vi "Make Defect Pair (old).vi"() -> ()   [LabVIEW 2010]
uses:
  <vilib>/Analysis/NI_AALPro.lvlib
  <vilib>/Analysis/_algsub.llb/Real Vector Norm.vi
panel:
  out "Atoms to Add":cluster{"Species":string, "Position":dbl[]}[](array[cluster])
  out "Atoms to remove":T1(array[cluster])
  out "Defected Structure":T2={"Structure Name"="Gamma8_64atom", "Lattice vector a"=[13.21796569573, 0.0, 0.0], "Lattice vector b"=[0.0, 13.21796569573, 0.0], "Lattice vector c"=[0.0, 0.0, 13.21796569573], "Atoms Array"=[{"Atom Name"="Cd", "Positions (Direct)"=[[0.0, 0.0, 0.0], [0.0, 0.0, 0.5], [0.0, 0.5, 0.0], [0.0, 0.5, 0.5], [0.5, 0.0, 0.0], [0.5, 0.0, 0.5], [0.5, 0.5, 0.0], [0.5, 0.5, 0.5], [0.0, 0.25, 0.25], [0.0, 0.25, 0.75], [0.0, 0.75, 0.25], [0.0, 0.75, 0.75], [0.5, 0.25, 0.25], [0.5, 0.25, 0.75], [0.5, 0.75, 0.25], [0.5, 0.75, 0.75], [0.25, 0.0, 0.25], [0.25, 0.0, 0.75], [0.25, 0.5, 0.25], [0.25, 0.5, 0.75], [0.75, 0.0, 0.25], [0.75, 0.0, 0.75], [0.75, 0.5, 0.25], [0.75, 0.5, 0.75], [0.25, 0.25, 0.0], [0.25, 0.25, 0.5], [0.25, 0.75, 0.0], [0.25, 0.75, 0.5], [0.75, 0.25, 0.0], [0.75, 0.25, 0.5], [0.75, 0.75, 0.0], [0.75, 0.75, 0.5]], "Positions (Cartesian)"=[[0.0, 0.0, 0.0], [0.0, 0.0, 6.608982847865], [0.0, 6.608982847865, 0.0], [0.0, 6.608982847865, 6.608982847865], [6.608982847865, 0.0, 0.0], [6.608982847865, 0.0, 6.608982847865], [6.608982847865, 6.608982847865, 0.0], [6.608982847865, 6.608982847865, 6.608982847865], [0.0, 3.3044914239325, 3.3044914239325], [0.0, 3.3044914239325, 9.913474271797499], [0.0, 9.913474271797499, 3.3044914239325], [0.0, 9.913474271797499, 9.913474271797499], [6.608982847865, 3.3044914239325, 3.3044914239325], [6.608982847865, 3.3044914239325, 9.913474271797499], [6.608982847865, 9.913474271797499, 3.3044914239325], [6.608982847865, 9.913474271797499, 9.913474271797499], [3.3044914239325, 0.0, 3.3044914239325], [3.3044914239325, 0.0, 9.913474271797499], [3.3044914239325, 6.608982847865, 3.3044914239325], [3.3044914239325, 6.608982847865, 9.913474271797499], [9.913474271797499, 0.0, 3.3044914239325], [9.913474271797499, 0.0, 9.913474271797499], [9.913474271797499, 6.608982847865, 3.3044914239325], [9.913474271797499, 6.608982847865, 9.913474271797499], [3.3044914239325, 3.3044914239325, 0.0], [3.3044914239325, 3.3044914239325, 6.608982847865], [3.3044914239325, 9.913474271797499, 0.0], [3.3044914239325, 9.913474271797499, 6.608982847865], [9.913474271797499, 3.3044914239325, 0.0], [9.913474271797499, 3.3044914239325, 6.608982847865], [9.913474271797499, 9.913474271797499, 0.0], [9.913474271797499, 9.913474271797499, 6.608982847865]]}, {"Atom Name"="Te", "Positions (Direct)"=[[0.125, 0.125, 0.125], [0.125, 0.125, 0.625], [0.125, 0.625, 0.125], [0.125, 0.625, 0.625], [0.625, 0.125, 0.125], [0.625, 0.125, 0.625], [0.625, 0.625, 0.125], [0.625, 0.625, 0.625], [0.375, 0.375, 0.125], [0.375, 0.375, 0.625], [0.375, 0.875, 0.125], [0.375, 0.875, 0.625], [0.875, 0.375, 0.125], [0.875, 0.375, 0.625], [0.875, 0.875, 0.125], [0.875, 0.875, 0.625], [0.375, 0.125, 0.375], [0.375, 0.125, 0.875], [0.375, 0.625, 0.375], [0.375, 0.625, 0.875], [0.875, 0.125, 0.375], [0.875, 0.125, 0.875], [0.875, 0.625, 0.375], [0.875, 0.625, 0.875], [0.125, 0.375, 0.375], [0.125, 0.375, 0.875], [0.125, 0.875, 0.375], [0.125, 0.875, 0.875], [0.625, 0.375, 0.375], [0.625, 0.375, 0.875], [0.625, 0.875, 0.375], [0.625, 0.875, 0.875]], "Positions (Cartesian)"=[[1.65224571196625, 1.65224571196625, 1.65224571196625], [1.65224571196625, 1.65224571196625, 8.261228559831249], [1.65224571196625, 8.261228559831249, 1.65224571196625], [1.65224571196625, 8.261228559831249, 8.261228559831249], [8.261228559831249, 1.65224571196625, 1.65224571196625], [8.261228559831249, 1.65224571196625, 8.261228559831249], [8.261228559831249, 8.261228559831249, 1.65224571196625], [8.261228559831249, 8.261228559831249, 8.261228559831249], [4.9567371358987495, 4.9567371358987495, 1.65224571196625], [4.9567371358987495, 4.9567371358987495, 8.261228559831249], [4.9567371358987495, 11.56571998376375, 1.65224571196625], [4.9567371358987495, 11.56571998376375, 8.261228559831249], [11.56571998376375, 4.9567371358987495, 1.65224571196625], [11.56571998376375, 4.9567371358987495, 8.261228559831249], [11.56571998376375, 11.56571998376375, 1.65224571196625], [11.56571998376375, 11.56571998376375, 8.261228559831249], [4.9567371358987495, 1.65224571196625, 4.9567371358987495], [4.9567371358987495, 1.65224571196625, 11.56571998376375], [4.9567371358987495, 8.261228559831249, 4.9567371358987495], [4.9567371358987495, 8.261228559831249, 11.56571998376375], [11.56571998376375, 1.65224571196625, 4.9567371358987495], [11.56571998376375, 1.65224571196625, 11.56571998376375], [11.56571998376375, 8.261228559831249, 4.9567371358987495], [11.56571998376375, 8.261228559831249, 11.56571998376375], [1.65224571196625, 4.9567371358987495, 4.9567371358987495], [1.65224571196625, 4.9567371358987495, 11.56571998376375], [1.65224571196625, 11.56571998376375, 4.9567371358987495], [1.65224571196625, 11.56571998376375, 11.56571998376375], [8.261228559831249, 4.9567371358987495, 4.9567371358987495], [8.261228559831249, 4.9567371358987495, 11.56571998376375], [8.261228559831249, 11.56571998376375, 4.9567371358987495], [8.261228559831249, 11.56571998376375, 11.56571998376375]]}], "# of atoms"=64}
  out "Defect Options":T3(array[cluster])=[{"Position"=[1.65224571196625, 1.65224571196625, 1.65224571196625], "Distance from 1"=2.8617735197133576, "Index"=0}, {"Position"=[4.9567371358987495, 4.9567371358987495, 1.65224571196625], "Distance from 1"=7.201972088359295, "Index"=8}, {"Position"=[4.9567371358987495, 1.65224571196625, 4.9567371358987495], "Distance from 1"=7.201972088359295, "Index"=16}, {"Position"=[1.65224571196625, 4.9567371358987495, 4.9567371358987495], "Distance from 1"=7.201972088359295, "Index"=24}]
  in  "Defect 2":cluster{"Species":string, "Defect Type":string}={"Species"="Te", "Defect Type"="Vacancy"}
  in  "Defect 1":cluster{"Species":string, "Defect Type":string}={"Species"="Cd", "Defect Type"="Vacancy"}
  in  "Defect 1 Atom Index":i32
  in  "Current Atomic Structure":T2={"Structure Name"="Gamma8_64atom", "Lattice vector a"=[13.21796569573, 0.0, 0.0], "Lattice vector b"=[0.0, 13.21796569573, 0.0], "Lattice vector c"=[0.0, 0.0, 13.21796569573], "Atoms Array"=[{"Atom Name"="Cd", "Positions (Direct)"=[[0.0, 0.0, 0.0], [0.0, 0.0, 0.5], [0.0, 0.5, 0.0], [0.0, 0.5, 0.5], [0.5, 0.0, 0.0], [0.5, 0.0, 0.5], [0.5, 0.5, 0.0], [0.5, 0.5, 0.5], [0.0, 0.25, 0.25], [0.0, 0.25, 0.75], [0.0, 0.75, 0.25], [0.0, 0.75, 0.75], [0.5, 0.25, 0.25], [0.5, 0.25, 0.75], [0.5, 0.75, 0.25], [0.5, 0.75, 0.75], [0.25, 0.0, 0.25], [0.25, 0.0, 0.75], [0.25, 0.5, 0.25], [0.25, 0.5, 0.75], [0.75, 0.0, 0.25], [0.75, 0.0, 0.75], [0.75, 0.5, 0.25], [0.75, 0.5, 0.75], [0.25, 0.25, 0.0], [0.25, 0.25, 0.5], [0.25, 0.75, 0.0], [0.25, 0.75, 0.5], [0.75, 0.25, 0.0], [0.75, 0.25, 0.5], [0.75, 0.75, 0.0], [0.75, 0.75, 0.5]], "Positions (Cartesian)"=[[0.0, 0.0, 0.0], [0.0, 0.0, 6.608982847865], [0.0, 6.608982847865, 0.0], [0.0, 6.608982847865, 6.608982847865], [6.608982847865, 0.0, 0.0], [6.608982847865, 0.0, 6.608982847865], [6.608982847865, 6.608982847865, 0.0], [6.608982847865, 6.608982847865, 6.608982847865], [0.0, 3.3044914239325, 3.3044914239325], [0.0, 3.3044914239325, 9.913474271797499], [0.0, 9.913474271797499, 3.3044914239325], [0.0, 9.913474271797499, 9.913474271797499], [6.608982847865, 3.3044914239325, 3.3044914239325], [6.608982847865, 3.3044914239325, 9.913474271797499], [6.608982847865, 9.913474271797499, 3.3044914239325], [6.608982847865, 9.913474271797499, 9.913474271797499], [3.3044914239325, 0.0, 3.3044914239325], [3.3044914239325, 0.0, 9.913474271797499], [3.3044914239325, 6.608982847865, 3.3044914239325], [3.3044914239325, 6.608982847865, 9.913474271797499], [9.913474271797499, 0.0, 3.3044914239325], [9.913474271797499, 0.0, 9.913474271797499], [9.913474271797499, 6.608982847865, 3.3044914239325], [9.913474271797499, 6.608982847865, 9.913474271797499], [3.3044914239325, 3.3044914239325, 0.0], [3.3044914239325, 3.3044914239325, 6.608982847865], [3.3044914239325, 9.913474271797499, 0.0], [3.3044914239325, 9.913474271797499, 6.608982847865], [9.913474271797499, 3.3044914239325, 0.0], [9.913474271797499, 3.3044914239325, 6.608982847865], [9.913474271797499, 9.913474271797499, 0.0], [9.913474271797499, 9.913474271797499, 6.608982847865]]}, {"Atom Name"="Te", "Positions (Direct)"=[[0.125, 0.125, 0.125], [0.125, 0.125, 0.625], [0.125, 0.625, 0.125], [0.125, 0.625, 0.625], [0.625, 0.125, 0.125], [0.625, 0.125, 0.625], [0.625, 0.625, 0.125], [0.625, 0.625, 0.625], [0.375, 0.375, 0.125], [0.375, 0.375, 0.625], [0.375, 0.875, 0.125], [0.375, 0.875, 0.625], [0.875, 0.375, 0.125], [0.875, 0.375, 0.625], [0.875, 0.875, 0.125], [0.875, 0.875, 0.625], [0.375, 0.125, 0.375], [0.375, 0.125, 0.875], [0.375, 0.625, 0.375], [0.375, 0.625, 0.875], [0.875, 0.125, 0.375], [0.875, 0.125, 0.875], [0.875, 0.625, 0.375], [0.875, 0.625, 0.875], [0.125, 0.375, 0.375], [0.125, 0.375, 0.875], [0.125, 0.875, 0.375], [0.125, 0.875, 0.875], [0.625, 0.375, 0.375], [0.625, 0.375, 0.875], [0.625, 0.875, 0.375], [0.625, 0.875, 0.875]], "Positions (Cartesian)"=[[1.65224571196625, 1.65224571196625, 1.65224571196625], [1.65224571196625, 1.65224571196625, 8.261228559831249], [1.65224571196625, 8.261228559831249, 1.65224571196625], [1.65224571196625, 8.261228559831249, 8.261228559831249], [8.261228559831249, 1.65224571196625, 1.65224571196625], [8.261228559831249, 1.65224571196625, 8.261228559831249], [8.261228559831249, 8.261228559831249, 1.65224571196625], [8.261228559831249, 8.261228559831249, 8.261228559831249], [4.9567371358987495, 4.9567371358987495, 1.65224571196625], [4.9567371358987495, 4.9567371358987495, 8.261228559831249], [4.9567371358987495, 11.56571998376375, 1.65224571196625], [4.9567371358987495, 11.56571998376375, 8.261228559831249], [11.56571998376375, 4.9567371358987495, 1.65224571196625], [11.56571998376375, 4.9567371358987495, 8.261228559831249], [11.56571998376375, 11.56571998376375, 1.65224571196625], [11.56571998376375, 11.56571998376375, 8.261228559831249], [4.9567371358987495, 1.65224571196625, 4.9567371358987495], [4.9567371358987495, 1.65224571196625, 11.56571998376375], [4.9567371358987495, 8.261228559831249, 4.9567371358987495], [4.9567371358987495, 8.261228559831249, 11.56571998376375], [11.56571998376375, 1.65224571196625, 4.9567371358987495], [11.56571998376375, 1.65224571196625, 11.56571998376375], [11.56571998376375, 8.261228559831249, 4.9567371358987495], [11.56571998376375, 8.261228559831249, 11.56571998376375], [1.65224571196625, 4.9567371358987495, 4.9567371358987495], [1.65224571196625, 4.9567371358987495, 11.56571998376375], [1.65224571196625, 11.56571998376375, 4.9567371358987495], [1.65224571196625, 11.56571998376375, 11.56571998376375], [8.261228559831249, 4.9567371358987495, 4.9567371358987495], [8.261228559831249, 4.9567371358987495, 11.56571998376375], [8.261228559831249, 11.56571998376375, 4.9567371358987495], [8.261228559831249, 11.56571998376375, 11.56571998376375]]}], "# of atoms"=64}
  in  "Maximum Distnce":dbl=8.0
  in  "Minimum Distance":dbl
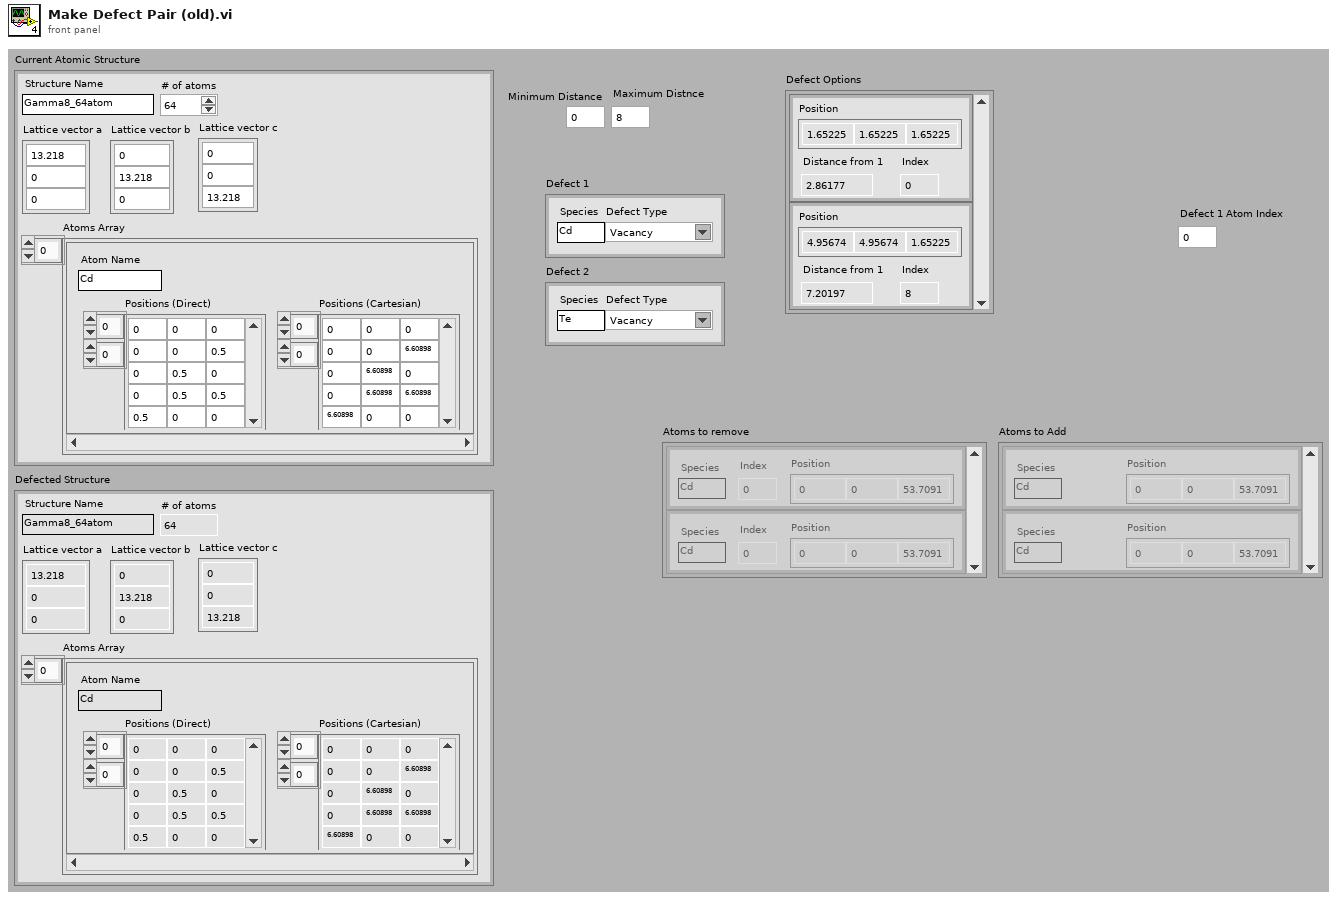
[diagram p1: front panel]
types:
  T1 = cluster{"Species":string, "Index":dbl, "Position":dbl[]}[]
  T2 = cluster{"Structure Name":string, "Lattice vector a":dbl[], "Lattice vector b":dbl[], "Lattice vector c":dbl[], "Atoms Array":cluster{"Atom Name":string, "Positions (Direct)":dbl[][], "Positions (Cartesian)":dbl[][]}[], "# of atoms":i32}
  T3 = cluster{"Position":dbl[], "Distance from 1":dbl, "Index":i32}[]
  T4 = cluster{"Positions (Cartesian)":dbl[], "norm":dbl, i32}[]
  T5 = cluster{"Atom Name":string, "Positions (Direct)":dbl[][], "Positions (Cartesian)":dbl[][]}[]
  T6 = cluster{"Species":string, "Defect 1 Atom Index":i32, "Positions (Cartesian)":dbl[]}
  T7 = cluster{"Atom Name":string, "Defect 1 Atom Index":i32, "Positions (Cartesian)":dbl[]}
  T8 = cluster{"Species":string, "Positions (Cartesian)":dbl[]}
  T9 = cluster{"Positions (Cartesian)":dbl[], "norm":dbl, i32}
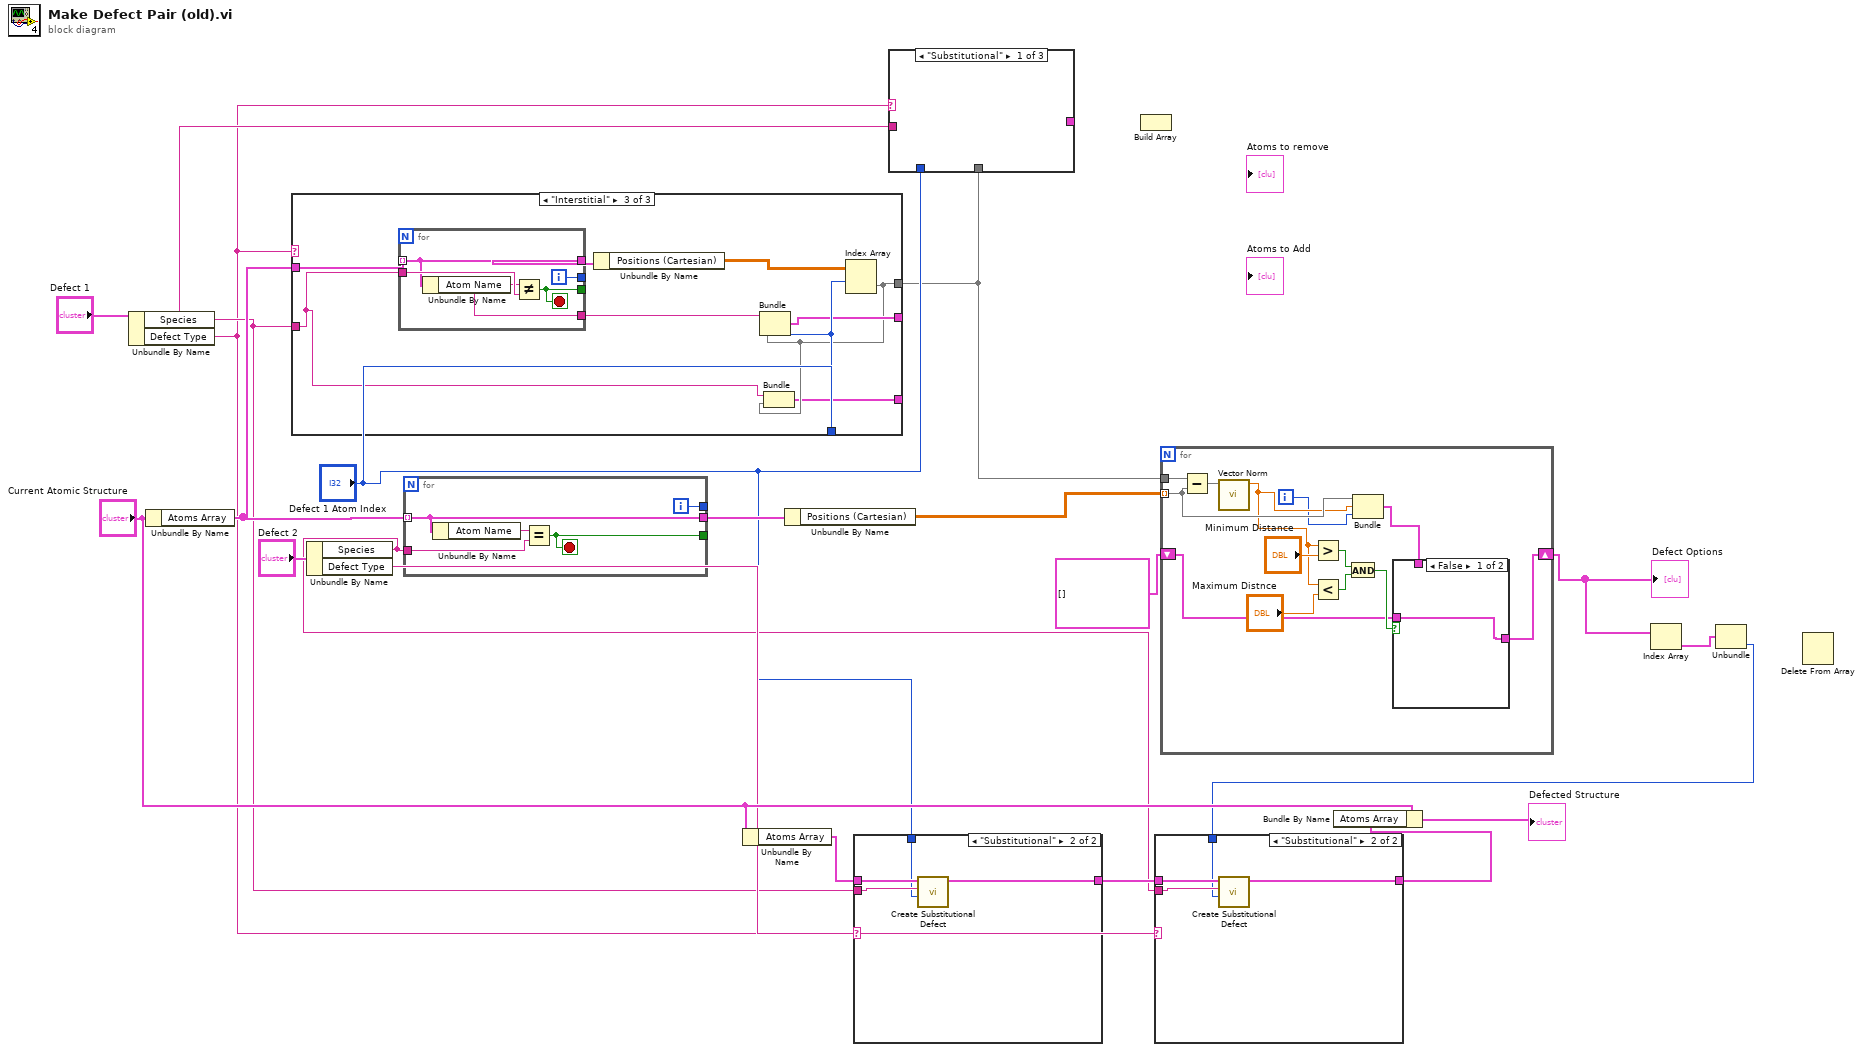
[diagram p0: block diagram]
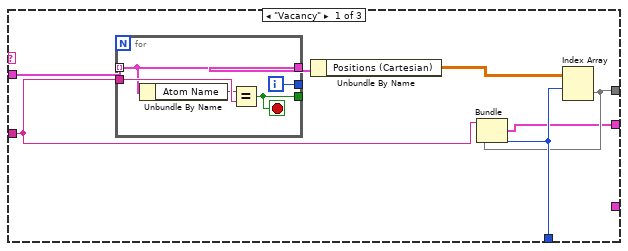
[diagram p2: hidden frame]
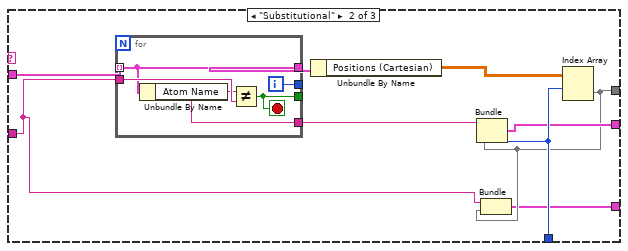
[diagram p3: hidden frame]
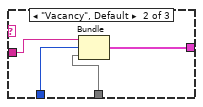
[diagram p4: hidden frame]
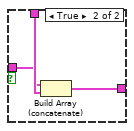
[diagram p8: hidden frame]
diagram:
  n1 = Unbundle By Name("Defect 1") -> ("Species"=w4:string, "Defect Type"=w1:string)
  n2 = Unbundle By Name("Current Atomic Structure") -> ("Atoms Array"=w20:T5)
  n3 = case shown="\"Interstitial\"" w1 {
    tunnel: w20 -> [w27 w41 w55]
    tunnel: w4 -> [w24 w35 w49]
    tunnel: "Defect 1 Atom Index" -> [w23 w38 w52]
    tunnel: [w22 w34 w48] -> w2
    tunnel: [w21 w37 w51] -> _
    tunnel: [_ w33 w47] -> _
    frame "Vacancy" {
      n4 = for {
        tunnel: w27 -> [w28] mode=indexing
        tunnel: w24 -> [w32]
        tunnel: [w30] -> _
        tunnel: [w29] -> _
        tunnel: [w28] -> w26
        i -> [w30]
        stop <- w29 stop-if-true
        n5 = Unbundle By Name(w28) -> ("Atom Name"=w31:string)
        n6 = Equal?(x=w31, y=w32) -> (x = y?=w29:bool)
      }
      n7 = Unbundle By Name(w26) -> ("Positions (Cartesian)"=w25:dbl[][])
      n8 = Index Array(array=w25, index (row)=w23) -> (element=w22:dbl[])  [unwired: 1 in]
      n9 = Bundle("Species"=w24, "Defect 1 Atom Index"=w23, "Positions (Cartesian)"=w22) -> (w21:T6)  [unwired: 1 in]
    }
    frame "Substitutional" {
      n10 = for {
        tunnel: w41 -> [w43] mode=indexing
        tunnel: w35 -> [w46]
        tunnel: [w45] -> _
        tunnel: [w44] -> _
        tunnel: [w43] -> w40
        tunnel: [w42] -> w36
        i -> [w45]
        stop <- w44 stop-if-true
        n11 = Unbundle By Name(w43) -> ("Atom Name"=w42:string)
        n12 = Not Equal?(x=w42, y=w46) -> (x != y?=w44:bool)
      }
      n13 = Unbundle By Name(w40) -> ("Positions (Cartesian)"=w39:dbl[][])
      n14 = Index Array(array=w39, index (row)=w38) -> (element=w34:dbl[])  [unwired: 1 in]
      n15 = Bundle("Atom Name"=w36, "Defect 1 Atom Index"=w38, "Positions (Cartesian)"=w34) -> (w37:T7)  [unwired: 1 in]
      n16 = Bundle("Species"=w35, "Positions (Cartesian)"=w34) -> (w33:T8)  [unwired: 1 in]
    }
    frame "Interstitial" {
      n17 = for {
        tunnel: w55 -> [w57] mode=indexing
        tunnel: w49 -> [w60]
        tunnel: [w59] -> _
        tunnel: [w58] -> _
        tunnel: [w57] -> w54
        tunnel: [w56] -> w50
        i -> [w59]
        stop <- w58 stop-if-true
        n18 = Unbundle By Name(w57) -> ("Atom Name"=w56:string)
        n19 = Not Equal?(x=w56, y=w60) -> (x != y?=w58:bool)
      }
      n20 = Unbundle By Name(w54) -> ("Positions (Cartesian)"=w53:dbl[][])
      n21 = Index Array(array=w53, index (row)=w52) -> (element=w48:dbl[])  [unwired: 1 in]
      n22 = Bundle("Atom Name"=w50, "Defect 1 Atom Index"=w52, "Positions (Cartesian)"=w48) -> (w51:T7)  [unwired: 1 in]
      n23 = Bundle("Species"=w49, "Positions (Cartesian)"=w48) -> (w47:T8)  [unwired: 1 in]
    }
  }
  n24 = Unbundle By Name("Defect 2") -> ("Species"=w7:string, "Defect Type"=w8:string)
  n25 = for {
    tunnel: w20 -> [w61] mode=indexing
    tunnel: w7 -> [w65]
    tunnel: [w63] -> _
    tunnel: [w62] -> _
    tunnel: [w61] -> w18
    i -> [w63]
    stop <- w62 stop-if-true
    n26 = Unbundle By Name(w61) -> ("Atom Name"=w64:string)
    n27 = Equal?(x=w64, y=w65) -> (x = y?=w62:bool)
  }
  n28 = Unbundle By Name("Current Atomic Structure") -> ("Atoms Array"=w10:T5)
  n29 = Unbundle By Name(w18) -> ("Positions (Cartesian)"=w17:dbl[][])
  n30 = case shown="\"Substitutional\"" w1 {
    tunnel: w10 -> [_ w69]
    tunnel: [_ w68] -> w9
    tunnel: w4 -> [_ w67]
    tunnel: "Defect 1 Atom Index" -> [_ w66]
    frame "False", Default {
    }
    frame "Substitutional" {
      n31 = call "Create Substitutional Defect.vi"("Indecies of replacement"=w66, "Atom Species"=w67, "Atoms Array"=w69) -> ("Atoms array with substitution"=w68:T5)  [unwired: 8 in]
    }
  }
  n32 = case shown="\"Substitutional\"" w1 {
    tunnel: w4 -> [_ w73 _]
    tunnel: "Defect 1 Atom Index" -> [_ w72 _]
    tunnel: w2 -> [_ w71 _]
    tunnel: [_ w70 _] -> _
    frame "Substitutional" {
    }
    frame "Vacancy", Default {
      n33 = Bundle("Species"=w73, "Defect 1 Atom Index"=w72, "Positions (Cartesian)"=w71) -> (w70:T6)  [unwired: 1 in]
    }
    frame "Interstitial" {
    }
  }
  n34 = Build Array() -> ()  [unwired: 2 in, 1 out]
  n35 = for {
    tunnel: w17 -> [w79] mode=indexing
    tunnel: w2 -> [w86]
    shift-right: [w75] -> w15
    shift-left: T4 [] -> [w74]
    i -> [w77]
    n36 = Subtract(x=w86, y=w79) -> (x-y=w85:dbl[])
    n37 = call-poly <vilib>:"Vector Norm.vi"("Input Vector"=w85) -> ("norm"=w78:dbl)  [unwired: 9 in, 1 out]
    n38 = Greater?(x=w78, y="Minimum Distance") -> (0:w82:bool)
    n39 = Less?(x=w78, y="Maximum Distnce") -> (x < y?=w81:bool)
    n40 = And(x=w82, y=w81) -> (x .and. y?=w80:bool)
    n41 = Bundle("Positions (Cartesian)"=w79, "norm"=w78, w77) -> (w76:T9)  [unwired: 1 in]
    n42 = case shown="False" w80 {
      tunnel: w76 -> [_ w90]
      tunnel: [w87 w89] -> w75
      tunnel: w74 -> [w87 w88]
      frame False {
      }
      frame True {
        n43 = Build Array (concatenate)(w88, w90) -> (w89:T4)
      }
    }
  }
  "Defect Options" <- w15
  n44 = Index Array(array=w15) -> (element=w14:T9)  [unwired: 1 in]
  n45 = Unbundle(w14) -> (w6:i32)  [unwired: 2 out]
  n46 = case shown="\"Substitutional\"" w8 {
    tunnel: w9 -> [_ w94]
    tunnel: [_ w93] -> w5
    tunnel: w7 -> [_ w92]
    tunnel: w6 -> [_ w91]
    frame "False", Default {
    }
    frame "Substitutional" {
      n47 = call "Create Substitutional Defect.vi"("Indecies of replacement"=w91, "Atom Species"=w92, "Atoms Array"=w94) -> ("Atoms array with substitution"=w93:T5)  [unwired: 8 in]
    }
  }
  n48 = Bundle By Name(cluster="Current Atomic Structure", "Atoms Array"=w5) -> (→"Defected Structure":T2)
  n49 = Delete From Array() -> ()  [unwired: 3 in, 2 out]
